vi "teststreamer client.vi"() -> ()   [LabVIEW 2016]
uses:
  dllwrapper/action complete event.ctl
  tls classes/connection creator/client connector/client connector.lvclass
  C:/Users/IEUser/Desktop/libasynclvtls/tls classes/connection creator/connection creator.lvclass
  tls classes/engine context/engine context.lvclass
  tls classes/connection/connection.lvclass
  tls classes/connection creator/connection creator.lvclass
  dllwrapper/async tls dl.lvlib
panel:
  out "bytes/s":dbl format="%#_9g"
  out "dt":dbl
  out "read bytes":i32
  in  "stop":bool
  out "error out":errorcluster
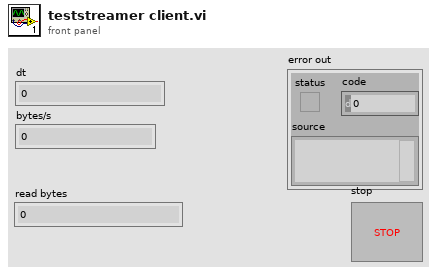
[diagram p1: front panel]
types:
  T1 = typedef "async tls dl.lvlib/action complete event.ctl" = cluster{"request ID":u32, "error code":i32, "error string":string}
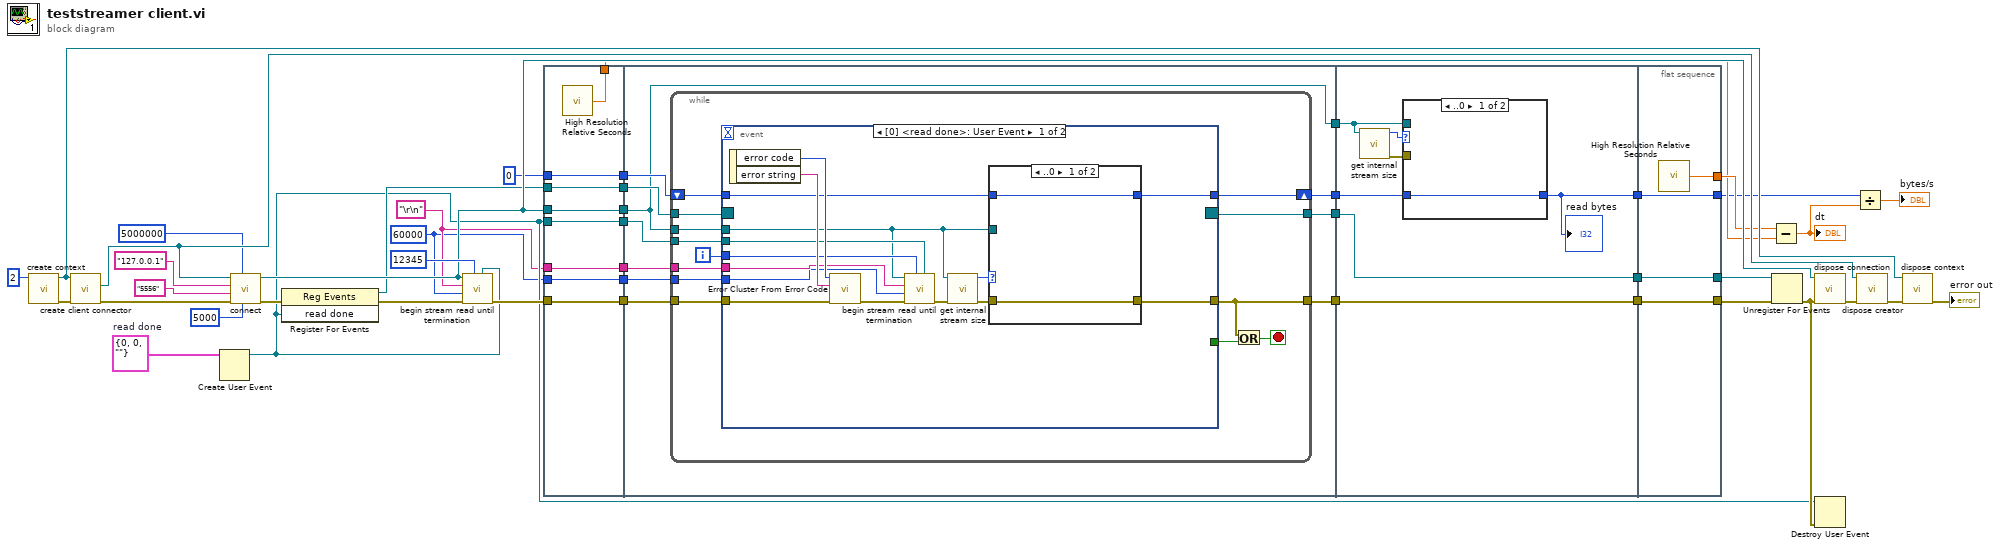
[diagram p0: block diagram]
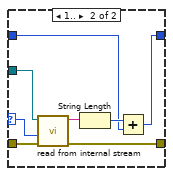
[diagram p2: hidden frame]
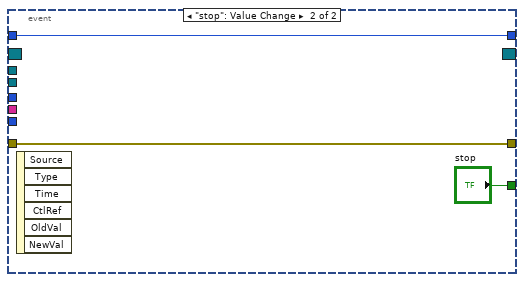
[diagram p3: hidden frame]
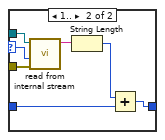
[diagram p4: hidden frame]
diagram:
  w10 = 60000 ("dimension size")
  w13 = "\r\n" ("termination")
  w30 = T1 {"request ID"=0, "error code"=0, "error string"=""}  # read done
  n1 = call "create context.vi"("thread count"=u64 2) -> ("error out"=w45:errorcluster, "engine context out"=w36:refnum<class "engine context.lvclass">)  [unwired: 9 in]
  n2 = call "create client connector.vi"("error in"=w45, "engine context in"=w36) -> ("error out"=w1:errorcluster, "client connector out"=w38:refnum<class "client connector.lvclass">)  [unwired: 8 in]
  n3 = Create User Event(user event datatype=w30) -> (user event=w17:refnum<user-event>)  [unwired: 1 in, 1 out]
  n4 = call "connect.vi"("timeout"=5000, "stream buffer size"=u64 5000000, "error in"=w1, "port"="5556", "host"="127.0.0.1", "client connector in"=w38) -> ("error out"=w28:errorcluster, "connection out"=w34:refnum<class "connection.lvclass">)  [unwired: 4 in]
  n5 = register-events(error in=w28, w17) -> (reference out=w26:refnum<event-registration>, error out=w27:errorcluster)  [unwired: 1 in]
  n6 = call "begin stream read until termination.vi"("event"=w17, "id"=u32 12345, "error in"=w27, "max bytes to read"=w10, "termination"=w13, "connection in"=w34) -> ("error out"=w40:errorcluster)  [unwired: 5 in]
  n7 = flat-sequence {
    tunnel: w17 -> [w49]
    tunnel: w26 -> [w50]
    tunnel: 0 -> [w51]
    tunnel: w34 -> [w52]
    tunnel: w40 -> [w53]
    tunnel: [w53] -> w24
    tunnel: [w52] -> w23
    tunnel: [w51] -> w22
    tunnel: [w50] -> w21
    tunnel: [w49] -> w20
    tunnel: [w48] -> w18
    tunnel: w13 -> [w47]
    tunnel: [w47] -> w12
    tunnel: [w46] -> w11
    tunnel: w10 -> [w46]
    tunnel: w24 -> [w63]
    tunnel: w23 -> [w54]
    tunnel: w22 -> [w60]
    tunnel: w21 -> [w59]
    tunnel: w20 -> [w58]
    tunnel: [w62] -> w9
    tunnel: [w61] -> w7
    tunnel: [w57] -> w5
    tunnel: w12 -> [w56]
    tunnel: w11 -> [w55]
    tunnel: [w54] -> w3
    tunnel: w9 -> [w107]
    tunnel: [w107] -> w8
    tunnel: w7 -> [w111]
    tunnel: [w111] -> w6
    tunnel: w5 -> [w106]
    tunnel: [w105] -> w4
    tunnel: w3 -> [w108]
    tunnel: [w122] -> w32
    tunnel: [w123] -> w33
    tunnel: w8 -> [w123]
    tunnel: w6 -> [w122]
    tunnel: [w121] -> w19
    tunnel: w4 -> [w120]
    tunnel: [w120] -> w16
    frame #0 {
      n8 = call <vilib>:"High Resolution Relative Seconds.vi"() -> ("relative seconds"=w48:dbl)
    }
    frame #1 {
      n9 = while {
        tunnel: w59 -> [w76]
        tunnel: w54 -> [w74]
        tunnel: [w70] -> w61
        tunnel: w63 -> [w75]
        tunnel: [w71] -> w62
        shift-right: [w68] -> w57
        shift-left: w60 -> [w69]
        tunnel: w58 -> [w67]
        tunnel: w56 -> [w65]
        tunnel: w55 -> [w64]
        i -> [w66]
        stop <- w72 stop-if-true
        n10 = event shown="[0] <read done>: User Event" {
          selector: w76 -> [_ _]
          dyn-events: [_ _] -> w70
          timeout: _ -> [_ _]
          tunnel: w75 -> [w91 w103]
          tunnel: [w79 w103] -> w71
          tunnel: w74 -> [w78 _]
          tunnel: [_ "stop"] -> w73
          tunnel: w69 -> [w81 w102]
          tunnel: [w80 w102] -> w68
          tunnel: w67 -> [w87 _]
          tunnel: w66 -> [w86 _]
          tunnel: w65 -> [w85 _]
          tunnel: w64 -> [w84 _]
          event User Event {
            n11 = event-data() -> ("error code"=w89:i32, "error string"=w88:string)  [unwired: 1 in]
            n12 = call <vilib>:"Error Cluster From Error Code.vi"("error in (no error)"=w91, "error message (\"\")"=w88, "error code (0)"=w89) -> ("error out"=w90:errorcluster)  [unwired: 6 in]
            n13 = call "begin stream read until termination.vi"("event"=w87, "id"=w86, "error in"=w90, "max bytes to read"=w84, "termination"=w85, "connection in"=w78) -> ("error out"=w77:errorcluster)  [unwired: 5 in]
            n14 = call "get internal stream size.vi"("error in"=w77, "connection in"=w78) -> ("error out"=w83:errorcluster, "size"=w82:u64)  [unwired: 8 in]
            n15 = case shown="..0" w82 {
              selector: w82 -> [_ w100]
              tunnel: w83 -> [w92 w101]
              tunnel: w81 -> [w93 w97]
              tunnel: [w93 w96] -> w80
              tunnel: [w92 w95] -> w79
              tunnel: w78 -> [_ w94]
              frame ..0 {
              }
              frame 1.. {
                n16 = call "read from internal stream.vi"("error in"=w101, "max length"=w100, "connection in"=w94) -> ("error out"=w95:errorcluster, "buffer"=w99:string)  [unwired: 7 in]
                n17 = String Length(string=w99) -> (length=w98:i32)
                n18 = Add(x=w98, y=w97) -> (x+y=w96:i32)
              }
            }
          }
          event "stop": Value Change {
            n19 = event-data() -> ()  [unwired: 1 in, 6 out]
          }
        }
        n20 = Or(x=w71, y=w73) -> (x .or. y?=w72:bool)
      }
    }
    frame #2 {
      n21 = call "get internal stream size.vi"("connection in"=w108) -> ("error out"=w109:errorcluster, "size"=w110:u64)  [unwired: 9 in]
      n22 = case shown="..0" w110 {
        selector: w110 -> [_ w117]
        tunnel: w109 -> [_ w116]
        tunnel: w108 -> [_ w115]
        tunnel: w106 -> [w112 w114]
        tunnel: [w112 w113] -> w105
        frame ..0 {
        }
        frame 1.. {
          n23 = call "read from internal stream.vi"("error in"=w116, "max length"=w117, "connection in"=w115) -> ("buffer"=w118:string)  [unwired: 7 in, 1 out]
          n24 = String Length(string=w118) -> (length=w119:i32)
          n25 = Add(x=w119, y=w114) -> (x+y=w113:i32)
        }
      }
      "read bytes" <- w105
    }
    frame #3 {
      n26 = call <vilib>:"High Resolution Relative Seconds.vi"() -> ("relative seconds"=w121:dbl)
    }
  }
  n27 = Subtract(x=w19, y=w18) -> (x-y=w15:dbl)
  "dt" <- w15
  n28 = Unregister For Events(event registration refnum=w32, error in=w33) -> (error out=w29:errorcluster)
  n29 = call "dispose connection.vi"("error in"=w29, "connection in"=w34) -> ("error out"=w39:errorcluster)  [unwired: 9 in]
  n30 = Destroy User Event(user event=w17, error in=w29) -> ()  [unwired: 1 out]
  n31 = Divide(x=w16, y=w15) -> (x/y=→"bytes/s":dbl)
  n32 = call "dispose creator.vi"("error in"=w39, "connection creator in"=w38) -> ("error out"=w37:errorcluster)  [unwired: 9 in]
  n33 = call "dispose context.vi"("error in"=w37, "engine context out"=w36) -> ("error out"=→"error out":errorcluster)  [unwired: 9 in]
